vi "MarkersTest_Plus.vi"() -> ()   [LabVIEW 2014]
uses:
  <userlib>/Nanonis Prog Interface V5/Nanonis Prog Interface.lvlib
panel:
  in  "Delete Last":bool
  in  "stop":bool
  in  "Show":bool
  in  "Delete All":bool
  in  "Text 2":string="X"
  in  "Draw Tip":bool
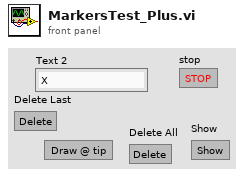
[diagram p1: front panel]
types:
  T1 = cluster{"X (m)":sgl, "Y (m)":sgl, "Text":string, "Color":u32, "Visible":bool}[]
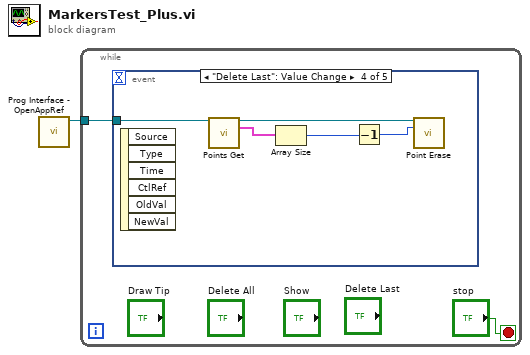
[diagram p0: block diagram]
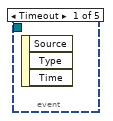
[diagram p2: hidden frame]
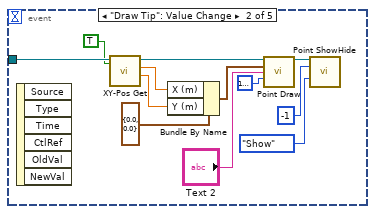
[diagram p3: hidden frame]
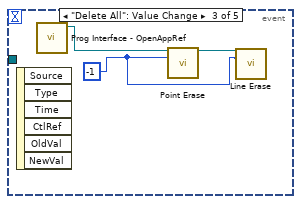
[diagram p4: hidden frame]
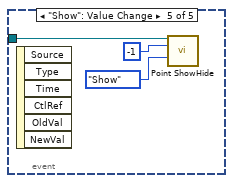
[diagram p5: hidden frame]
diagram:
  n1 = call <userlib>:"Prog Interface - OpenAppRef.vi"() -> ("Application reference"=w1:refnum<vi>)  [unwired: 6 in, 1 out]
  n2 = while {
    tunnel: w1 -> [w3]
    stop <- "stop" stop-if-true
    n3 = event shown="[3] \"Delete Last\": Value Change" {
      selector: _ -> [_ _ _ _ _]
      dyn-events: _ -> [_ _ _ _ _]
      timeout: _ -> [_ _ _ _ _]
      tunnel: w3 -> [_ w5 _ w21 w24]
      event Timeout {
        n4 = event-data() -> ()  [unwired: 1 in, 3 out]
      }
      event "Draw Tip": Value Change {
        n5 = event-data() -> ()  [unwired: 1 in, 6 out]
        n6 = call <userlib>:"XY-Pos Get.vi"("Wait for newest data (F=False)"=TRUE, "Application ref in"=w5) -> ("Y (m)"=w14:sgl, "X (m)"=w13:sgl, "Application ref out"=w15:refnum<vi>)  [unwired: 5 in, 1 out]
        n7 = Bundle By Name(cluster=cluster{"X (m)":sgl, "Y (m)":sgl} {"X (m)"=0.0, "Y (m)"=0.0} ("Point Coordinates"), "X (m)"=w13, "Y (m)"=w14) -> (w12:cluster{"X (m)":sgl, "Y (m)":sgl})
        n8 = call <userlib>:"Point Draw.vi"("Application ref in"=w15, "Point Coordinates"=w12, "Text"="Text 2", "Color"=u32 16777216) -> ("Application ref out"=w8:refnum<vi>)  [unwired: 10 in, 1 out]
        n9 = call <userlib>:"Point ShowHide.vi"("Application ref in"=w8, "Point index (-1=All points)"=-1, "Show/Hide"=enum16{"Show", "Hide"}."Show") -> ()  [unwired: 11 in, 2 out]
      }
      event "Delete All": Value Change {
        w16 = -1 ("Point index (-1=All points)")
        n10 = event-data() -> ()  [unwired: 1 in, 6 out]
        n11 = call <userlib>:"Prog Interface - OpenAppRef.vi"() -> ("Application reference"=w18:refnum<vi>)  [unwired: 6 in, 1 out]
        n12 = call <userlib>:"Point Erase.vi"("Application ref in"=w18, "Point index (-1=All points)"=w16) -> ("Application ref out"=w17:refnum<vi>)  [unwired: 12 in, 1 out]
        n13 = call <userlib>:"Line Erase.vi"("Application ref in"=w17, "Line index (-1=All lines)"=w16) -> ()  [unwired: 12 in, 2 out]
      }
      event "Delete Last": Value Change {
        n14 = event-data() -> ()  [unwired: 1 in, 6 out]
        n15 = call <userlib>:"Points Get.vi"("Application ref in"=w21) -> ("Application ref out"=w20:refnum<vi>, "Points"=w22:T1)  [unwired: 12 in, 1 out]
        n16 = Array Size(array=w22) -> (size(s)=w23:i32)
        n17 = Decrement(x=w23) -> (x-1=w19:i32)
        n18 = call <userlib>:"Point Erase.vi"("Application ref in"=w20, "Point index (-1=All points)"=w19) -> ()  [unwired: 12 in, 2 out]
      }
      event "Show": Value Change {
        n19 = event-data() -> ()  [unwired: 1 in, 6 out]
        n20 = call <userlib>:"Point ShowHide.vi"("Application ref in"=w24, "Point index (-1=All points)"=-1, "Show/Hide"=enum16{"Show", "Hide"}."Show") -> ()  [unwired: 11 in, 2 out]
      }
    }
  }
